vi "Check Object Lengths.vi"(8 "error in":errorcluster, 11 "objects in":T1[](array[typedef]) {"Object ID" format="%x"}) -> (0 "error out":errorcluster, 3 "objects out":T1[](array[typedef]) {"Object ID" format="%x"})   [LabVIEW 2015, in "Modbus Library.lvlib"]
doc: "Checks to ensure that all Modbus objects can fit within the length allowed by the Modbus protocol data unit and will throw an error if any object is longer than allowed. This check must be performed because objects may not be split across multiple data units, although a request for multiple objects can be split across multiple responses."
uses:
  Modbus Library.lvlib
  Data Model/Identification Parameters.ctl
  Data Model/Device Data Model.lvclass
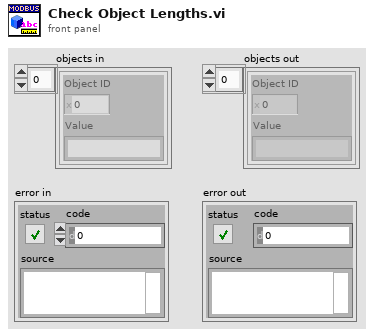
[diagram p1: front panel]
types:
  T1 = typedef "Modbus Library.lvlib/Device Data Model.lvclass/Identification Parameters.ctl" = cluster{"Object ID":u8, "Value":string}
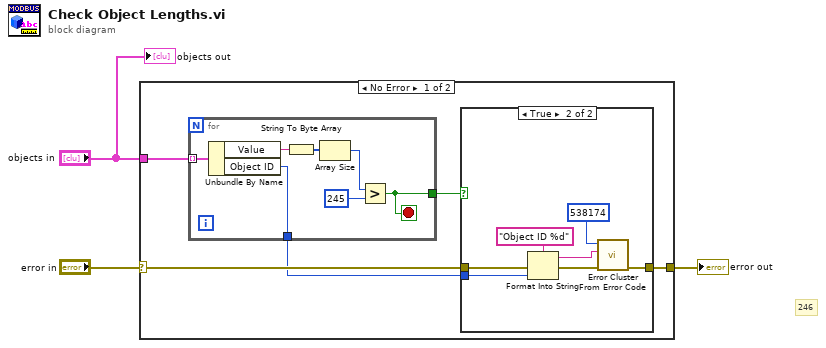
[diagram p0: block diagram]
diagram:
  # "246"
  n1 = case shown="No Error" "error in" {
    selector: "error in" -> [w6 w24]
    tunnel: [w5 w24] -> w2
    tunnel: "objects in" -> [w8 _]
    frame No Error {
      n2 = for {
        tunnel: w8 -> [w23] mode=indexing
        tunnel: [w18] -> w7
        tunnel: [w17] -> w4
        stop <- w18 stop-if-true
        n3 = Unbundle By Name(w23) -> ("Value"=w22:string, "Object ID"=w17:u8)
        n4 = String To Byte Array(string=w22) -> (unsigned byte array=w21:u8[])
        n5 = Array Size(array=w21) -> (size(s)=w20:i32)
        n6 = Greater?(x=w20, y=245) -> (0:w18:bool)
      }
      n7 = case shown="True" w7 {
        tunnel: w6 -> [w9 w14]
        tunnel: [w9 w16] -> w5
        tunnel: w4 -> [_ w11]
        frame False {
        }
        frame True {
          n8 = Format Into String(format string="Object ID %d", error in=w14, w11) -> (resulting string=w12:string, error out=w13:errorcluster)  [unwired: 1 in]
          n9 = call <vilib>:"Error Cluster From Error Code.vi"("error in (no error)"=w13, "error message (\"\")"=w12, "error code (0)"=538174) -> ("error out"=w16:errorcluster)  [unwired: 6 in]
        }
      }
    }
    frame Error {
    }
  }
  "error out" <- w2
  "objects out" <- "objects in"
